vi "Temperature.vi"() -> ()   [LabVIEW 2015]
uses:
  <vilib>/DAQmx/read.llb/DAQmx Read (Analog 1D DBL 1Chan NSamp).vi
  <vilib>/Analysis/baseanly.llb/Mean (DBL).vi
  <vilib>/DAQmx/create/channels.llb/DAQmx Create Channel (AI-Voltage-Basic).vi
  <vilib>/DAQmx/configure/timing.llb/DAQmx Timing (Sample Clock).vi
  <vilib>/DAQmx/miscellaneous.llb/DAQmx Fill In Error Info.vi
  <vilib>/Analysis/NI_AALBase.lvlib
panel:
  in  "Temp option":bool
  out "Temperature":dbl(graph)
  out "mean signal (V)":dbl format="%.3f"
  in  "exit":bool
  in  "Sampling rate":dbl=1000.0 format="%#.2f"
  in  "Physical channels":tag
  out "Signal":dbl[](graph)
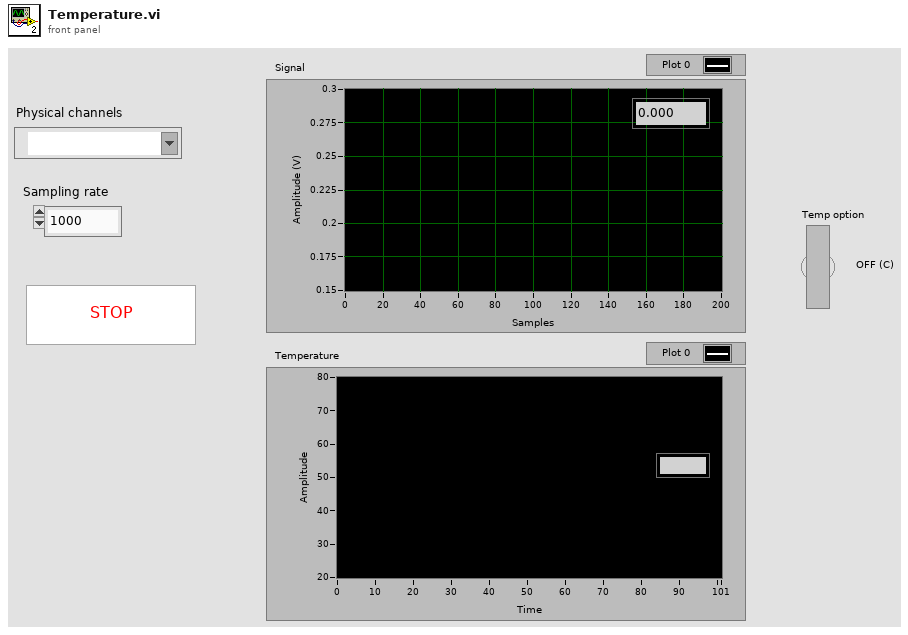
[diagram p1: front panel]
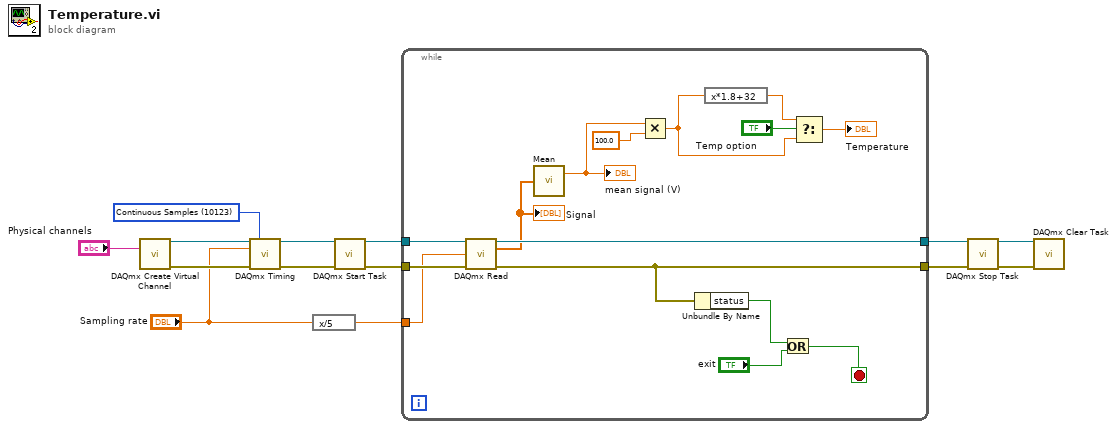
[diagram p0: block diagram]
diagram:
  w11 = 10123 items=["Finite Samples"=10178, "Continuous Samples"=10123, "Hardware Timed Single Point"=12522] ("sample mode")
  n1 = call-poly <vilib>:"DAQmx Create Virtual Channel.vi"("physical channels"="Physical channels") -> ("task out"=w14:refnum<k21>, "error out"=w13:errorcluster)  [unwired: 13 in]
  n2 = call-poly <vilib>:"DAQmx Timing.vi"("task/channels in"=w14, "sample mode"=w11, "rate"="Sampling rate", "error in"=w13) -> ("task out"=w6:refnum<k21>, "error out"=w9:errorcluster)  [unwired: 10 in]
  n3 = expression code="x/5"("Sampling rate") -> (w5:dbl)
  n4 = call <vilib>:"DAQmx Start Task.vi"("task/channels in"=w6, "error in"=w9) -> ("task out"=w7:refnum<k21>, "error out"=w8:errorcluster)  [unwired: 12 in]
  n5 = while {
    tunnel: w7 -> [w29]
    tunnel: [w28] -> w2
    tunnel: w8 -> [w27]
    tunnel: [w24] -> w3
    tunnel: w5 -> [w25]
    stop <- w21 stop-if-true
    n6 = call-poly <vilib>:"DAQmx Read.vi"("task/channels in"=w29, "number of samples per channel"=w25, "error in"=w27) -> ("task out"=w28:refnum<k21>, "data"=w26:dbl[], "error out"=w24:errorcluster)  [unwired: 10 in]
    "Signal" <- w26
    n7 = call-poly <vilib>:"Mean.vi"("X"=w26) -> ("mean"=w20:dbl)  [unwired: 1 out]
    "mean signal (V)" <- w20
    n8 = Multiply(x=w20, y=100.0) -> (x*y=w17:dbl)
    n9 = Unbundle By Name(w24) -> ("status"=w22:bool)
    n10 = expression code="x*1.8+32"(w17) -> (w18:dbl)
    n11 = Or(x=w22, y="exit") -> (x .or. y?=w21:bool)
    n12 = Select(t=w18, s="Temp option", f=w17) -> (s? t:f=→"Temperature":dbl)
  }
  n13 = call <vilib>:"DAQmx Stop Task.vi"("task/channels in"=w2, "error in"=w3) -> ("task out"=w1:refnum<k21>, "error out"=w4:errorcluster)  [unwired: 12 in]
  n14 = call <vilib>:"DAQmx Clear Task.vi"("task in"=w1, "error in"=w4) -> ()  [unwired: 13 in, 1 out]
